vi "Autonomous Independent.vi"() -> ()   [LabVIEW 2013]
doc: "This VI is called when autonomous begins, and will automatically be terminated when autonomous ends. You can carry out timed or sensor driven robot movement independently without needing to return to the caller."
uses:
  Robot Global Data.vi
  <vilib>/Rock Robotics/WPI/RobotDrive/WPI_RobotDriveGetSetRefNum.vi
panel:
  out "error  out":errorcluster
  # "Be sure to right-click and choose Data Operations>>Make Current Value default if you want to save the array values with the VI"
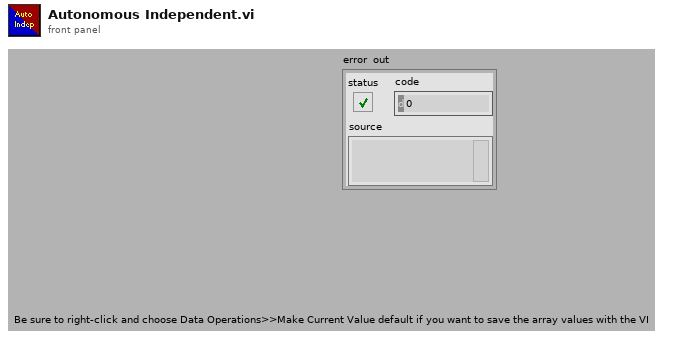
[diagram p1: front panel]
types:
  T1 = typedef "WPI_RobotDriveDevRef.ctl" = cluster{"DevStatus":errorcluster, "Motors[]":T2[], "Square Inputs":bool, "Max Output":dbl, "Isochronous":bool}
  T2 = typedef "WPI_MotorControlDeviceRef.ctl" = cluster{"DeviceStatus":errorcluster, "Type":enum16{"PWM", "CAN"}, "PWM":cluster{"Digital Module":T3, "PWM Channel":T4, "DeadBand":T5}, "CAN":cluster{"Device Number":u8, "Control Mode":T6, "Semaphore":T7, "Max Vout":dbl}, "Invert":bool, "TransformRef":T8, "InvTransformRef":T8}
  T3 = typedef "FPGA_TypedefDigitalModule.ctl" = enum16{"Digital Module 1", "Digital Module 2"}
  T4 = typedef "FPGA_DIOPWMChannel.ctl" = enum8{"PWM 1", "PWM 2", "PWM 3", "PWM 4", "PWM 5", "PWM 6", "PWM 7", "PWM 8", "PWM 9", "PWM 10", "Invalid"}
  T5 = typedef "WPI_PWMDeadband.ctl" = cluster{"Name":string, "maxPositivePwm":i32, "minPositivePwm":i32, "centerPwm":i32, "maxNegativePwm":i32, "minNegativePwm":i32, "angularRange":u16}
  T6 = typedef "WPI_CANJaguar_ControlMode.ctl" = enum8{"Percent VBus", "Current", "Speed", "Position", "Voltage"}
  T7 = typedef "Semaphore RefNum" = refnum<k1>
  T8 = typedef "WPI_PWMTransform_ConPane.ctl" = refnum<vi>
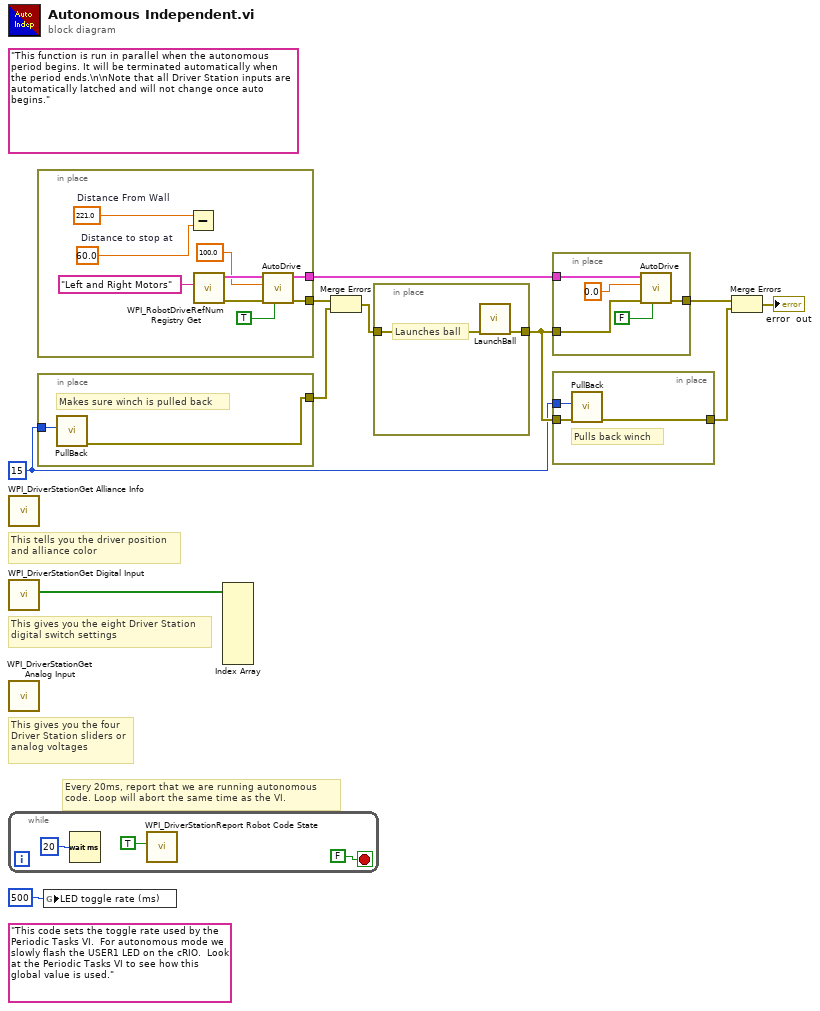
[diagram p0: block diagram]
diagram:
  w5 = 15 ("Timeout (s)")
  (unwired) "This code sets the toggle rate used by the Periodic Tasks VI.  For autonomous mode we slowly flash the USER1 LED on the cRIO.  Look at the Periodic Tasks VI to see how this global value is used."
  (unwired) "This function is run in parallel when the autonomous period begins. It will be terminated automatically when the period ends.\n\nNote that all Driver Station inputs are automatically latched and will not change once auto begins."
  # "Every 20ms, report that we are running autonomous\ncode. Loop will abort the same time as the VI."
  # "This tells you the driver position\nand alliance color"
  # "This gives you the eight Driver Station\ndigital switch settings"
  # "This gives you the four\nDriver Station sliders or\nanalog voltages"
  n1 = call <vilib>:"WPI_DriverStationGet Alliance Info.vi"() -> ()  [unwired: 12 out]
  n2 = call <vilib>:"WPI_DriverStationGet Digital Input.vi"() -> ("Driver Station Digital Input (1-8)"=w11:bool[])  [unwired: 11 out]
  n3 = call <vilib>:"WPI_DriverStationGet Analog Input.vi"() -> ()  [unwired: 12 out]
  n4 = while {
    stop <- FALSE stop-if-true
    n5 = Wait (ms)(milliseconds to wait=u32 20) -> ()  [unwired: 1 out]
    n6 = call <vilib>:"WPI_DriverStationReport Robot Code State.vi"("Autonomous"=TRUE) -> ()  [unwired: 10 in, 1 out]
  }
  n7 = in-place {
    in-place-border: [w18] -> w7
    in-place-border: [w17] -> w2
    w22 = 221.0  # Distance From Wall
    w23 = 60.0  # Distance to stop at
    n8 = Subtract(x=w22, y=w23) -> ()  [unwired: 1 out]
    n9 = call <vilib>:"WPI_RobotDriveRefNum Registry Get.vi"("refnum name"="Left and Right Motors") -> ("error out"=w19:errorcluster, "RobotDriveDevRef"=w20:T1)  [unwired: 9 in]
    n10 = call "AutoDrive.vi"("Forwards"=TRUE, "error in (no error)"=w19, "Input (inches)"=100.0, "RobotDriveDevRef"=w20) -> ("error out"=w17:errorcluster, "RobotDriveDevRef"=w18:T1)  [unwired: 6 in]
  }
  n11 = in-place {
    in-place-border: [w25] -> w9
    in-place-border: w5 -> [w24]
    # "Makes sure winch is pulled back"
    n12 = call "PullBack.vi"("Timeout (s)"=w24) -> ("error out"=w25:errorcluster)  [unwired: 10 in]
  }
  n13 = global write "Robot Global Data.vi" "LED toggle rate (ms)"(u32 500 ("LED ms toggle rate")) -> ()
  n14 = Index Array(array=w11) -> ()  [unwired: 8 in, 8 out]
  n15 = Merge Errors(w2, w9) -> (w8:errorcluster)
  n16 = in-place {
    in-place-border: w8 -> [w27]
    in-place-border: [w26] -> w6
    # "Launches ball"
    n17 = call "LaunchBall.vi"("error in (no error)"=w27) -> ("error out"=w26:errorcluster)  [unwired: 10 in]
  }
  n18 = in-place {
    in-place-border: w7 -> [w32]
    in-place-border: w6 -> [w31]
    in-place-border: [w30] -> w1
    n19 = call "AutoDrive.vi"("Forwards"=FALSE, "error in (no error)"=w31, "Input (inches)"=0.0, "RobotDriveDevRef"=w32) -> ("error out"=w30:errorcluster)  [unwired: 6 in, 1 out]
  }
  n20 = in-place {
    in-place-border: w6 -> [w35]
    in-place-border: w5 -> [w34]
    in-place-border: [w33] -> w4
    # "Pulls back winch"
    n21 = call "PullBack.vi"("error in (no error)"=w35, "Timeout (s)"=w34) -> ("error out"=w33:errorcluster)  [unwired: 9 in]
  }
  n22 = Merge Errors(w1, w4) -> (→"error  out":errorcluster)
